vi "plot_isoteric_chart.vi"(7 "W-Array in kg/kg (Input)":dbl[](array[numeric])=[0.01, 0.025, 0.1, 0.2, 0.3, 0.4, 0.5], 8 "Error (Input)":errorcluster, 9 "T_max in K (Input)":dbl=647.0, 10 "T_min in K (Input)":dbl=283.15, 11 "WorkingPair (Input)":T1={"no_iso"=1, "no_p_sat"=1, "path_db"="D:\\Driesel\\SorpLibLocal\\labview_wrapper\\data\\json\\sorpproplib.json", "wp_as"="silica gel pellet", "wp_st"="123", "wp_iso"="DubininArctan1", "wp_rf"="Water", "rf_rhol"="SaturatedLiquidDensity_EoS1", "no_rhol"=1, "rf_psat"="VaporPressure_EoS1"}) -> (0 "Error (Output)":errorcluster, 3 "Isosteres":cluster{dbl[], dbl[]}[](graph)=[{array[365 elements], array[365 elements]}, {array[365 elements], array[365 elements]}, {array[365 elements], array[365 elements]}, {array[365 elements], array[365 elements]}, {array[359 elements], array[359 elements]}, {array[289 elements], array[289 elements]}, {[-0.003531696980399082, -0.0035192679922576107, -0.0035069261792039282, -0.003494670627293378, -0.0034825004353125546, -0.00347041471455839, -0.003458412588621823, -0.0034464931931759437, -0.0034346556757685045, -0.0034228991956186893, -0.003411222923418046, -0.0033996260411354754, -0.0033881077418261903, -0.0033766672294445383, -0.0033653037186606094, -0.0033540164346805303, -0.003342804613070366, -0.003331667499583542, -0.003320604349991699, -0.0033096144299189145, -0.003298697014679202, -0.003287851389117212, -0.003277076847452073, -0.003266372693124286, -0.003255738238645613, -0.0032451728054518907, -0.0032346757237586934, -0.003224246332419797, -0.003213883978788366, -0.0032035880185808108, -0.003193357815743254, -0.0031831927423205475, -0.0031730921783277807, -0.003163055511624229, -0.0031530821377896896, -0.0031431714600031434, -0.0031333228889237038, -0.003123535842573794, -0.0031138097462245057, -0.003104144032283098, -0.0030945381401825778, -0.0030849915162733305, -0.0030755036137167465, -0.0030660738923808067, -0.0030567018187375823, -0.0030473868657626088, -0.0030381285128360932, -0.003028926245645919, -0.0030197795560924054, -0.0030106879421947915, -0.0030016509079994, -0.002992667963489451, -0.002983738624496494, -0.002974862412613417, -0.002966038855109002, -0.0029572674848440043, -0.0029485478401887074, -0.0029398794649419377, -0.0029312619082515023, -0.0029226947245360223, -0.002914177473408131, -0.002905709719599012, -0.0028972910328842532, -0.0028889209880109783, -0.0028805991646262425, -0.002872325147206664, -0.0028640985249892598, -0.00285591889190347, -0.002847785846504343, -0.002839698991906858, -0.002831657935721365, -0.002823662289990117, -0.002815711671124877, -0.002807805699845571, -0.0027999440011199778, -0.002792126204104426, -0.00278435194208548, -0.0027766208524226017, -0.0027689325764917627, -0.0027612867596299878, -0.002753683051080821, -0.002746121103940684, -0.002738600575106121, -0.0027311211252219036, -0.0027236824186299877, -0.0027162841233192994, -0.0027089259108763375, -0.00270160745643658, -0.00269432843863667, -0.002687088539567379, -0.0026798874447273215, -0.0026727248429774158, -0.0026656004264960682, -0.0026585138907350794], [995.6868807653667, 1065.5938991149683, 1139.8574391068994, 1218.7117814882488, 1302.401645095998, 1391.1825454296695, 1485.3211613320625, 1585.0957098471665, 1690.7963293242678, 1802.7254708382966, 1921.1982979968375, 2046.5430952054487, 2179.1016844642027, 2319.229850770136, 2467.297776201945, 2623.690482765518, 2788.808284081765, 2963.067246000752, 3146.899656229439, 3340.7545030642627, 3545.0979633235356, 3760.4138995790445, 3987.2043667916496, 4225.990128460064, 4477.311182398888, 4741.727296267391, 5019.818552977553, 5312.185906117583, 5619.451745534454, 5942.260473227631, 6281.279089715428, 6637.197791044433, 7010.730576623637, 7402.615868075008, 7813.6171393044415, 8244.523558008743, 8696.150638848858, 9169.34090853134, 9664.964583056706, 10183.920257407988, 10727.135607969129, 11295.568107981539, 11890.205756363213, 12512.067820236784, 13162.205591531703, 13841.703158047952, 14551.678189391017, 15293.282738212663, 16067.704057216224, 16876.165432412705, 17719.927033141066, 18600.286779396734, 19518.581227041646, 20476.186471504287, 21474.519070609156, 22515.036987215448, 23599.240552378036, 24728.673449789396, 25904.923722296717, 27129.624801339716, 28404.456560195467, 29731.146391970313, 31111.470313326685, 32547.25409499115, 34040.37442014383, 35592.76007185284, 37206.393150778495, 38883.310324442566, 40625.60410942416, 42435.42418792465, 44314.97876021472, 46266.53593457144, 48292.42515638591, 50395.03867823235, 52576.83307276827, 54840.33079046082, 57188.121764219315, 59622.8650631532, 62147.29059777922, 64764.20087914201, 67476.47283444299, 70287.0596819237, 73198.99286789467, 76215.38406897619, 79339.42726277668, 82574.40087043002, 85923.66997459781, 89390.68861675632, 92979.00217780344, 96692.2498462531, 100534.16717853813, 104508.58875619763, 108619.45094501246, 112870.79476144738]}, {[], []}])   [LabVIEW 2017]
panel:
  out "ID of temperature loop":i32=364
  # "Path to database"
  # "Name of sorbent"
  # "Name of sub-type of sorbent"
  # "Name of refrigerant"
  # "Name of isotherm"
  # "ID of isotherm"
  # "Name of calculation approach for vapor pressure"
  # "ID of vapor pressure equation"
  # "Name of calculation approach for liquid density"
  # "ID of liquid density equation"
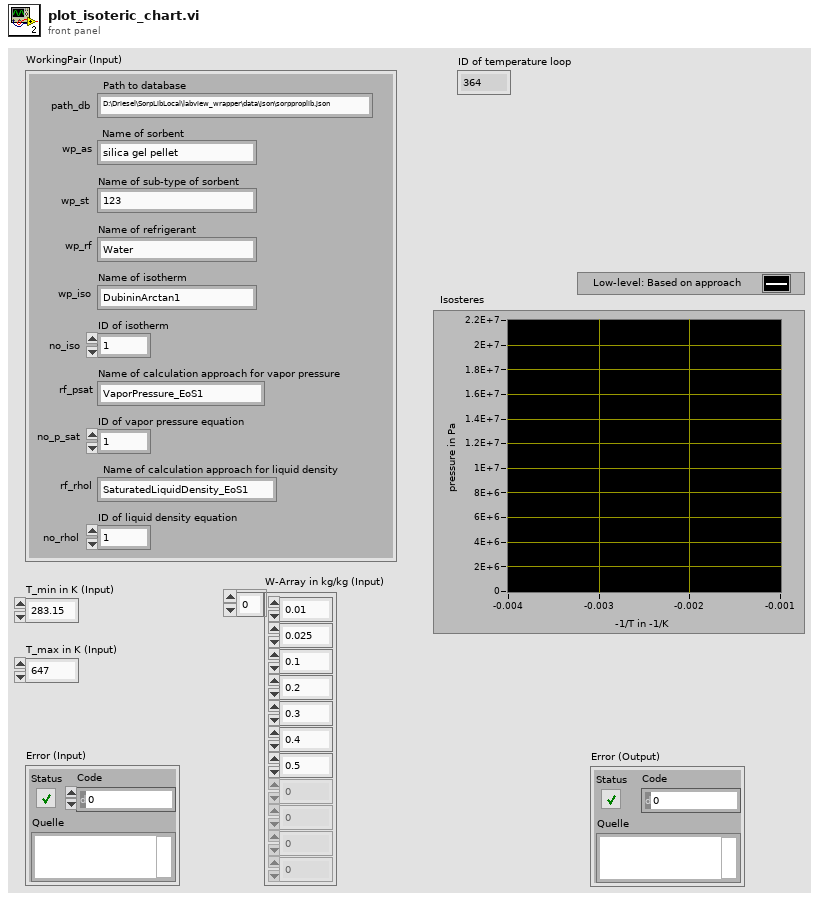
[diagram p1: front panel]
types:
  T1 = cluster{"no_iso":i32, "no_p_sat":i32, "path_db":string, "wp_as":string, "wp_st":string, "wp_iso":string, "wp_rf":string, "rf_rhol":string, "no_rhol":i32, "rf_psat":string}
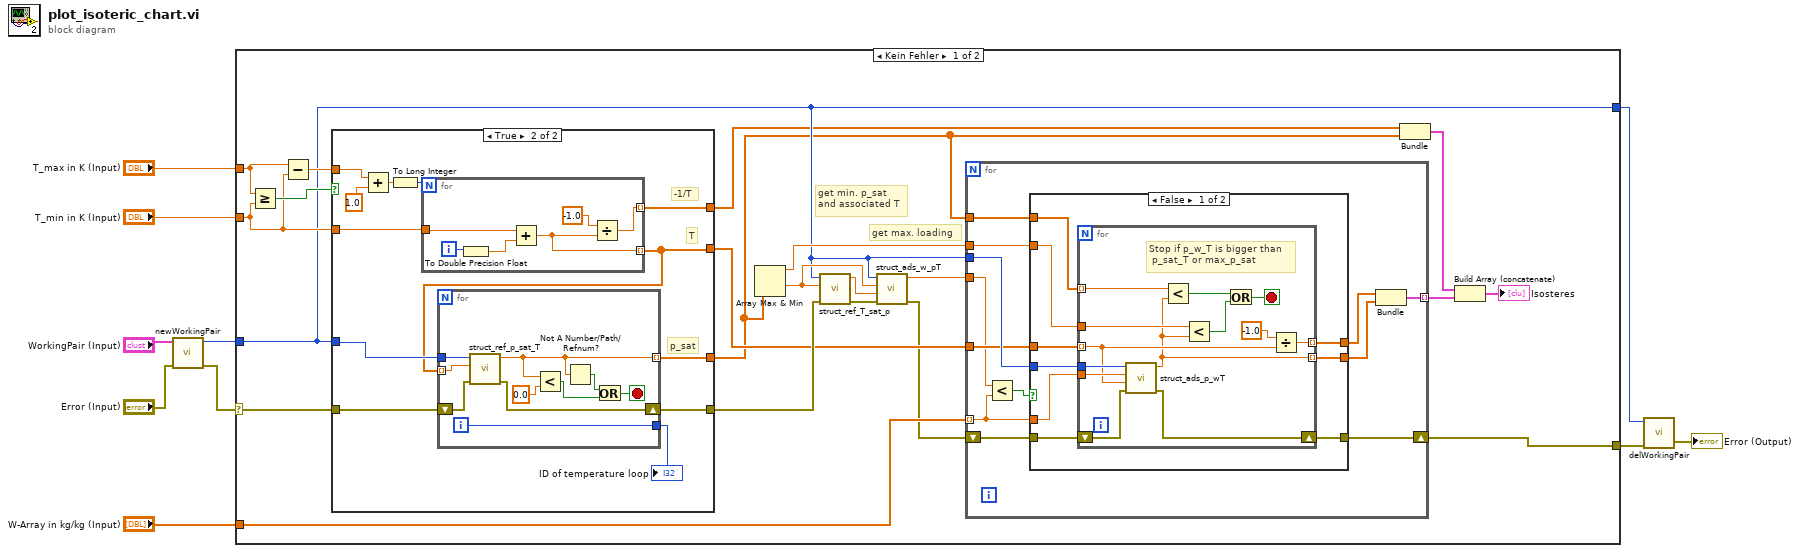
[diagram p0: block diagram]
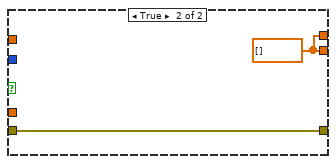
[diagram p2: hidden frame]
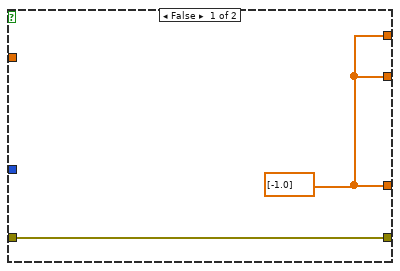
[diagram p3: hidden frame]
diagram:
  n1 = call "newWorkingPair.vi"("Error (Input)"="Error (Input)", "WorkingPair (Input)"="WorkingPair (Input)") -> ("Error (Output)"=w7:errorcluster, "workingPair"=w5:i64)  [unwired: 8 in]
  n2 = case shown="Kein Fehler" w7 {
    selector: w7 -> [w27 w99]
    tunnel: [w22 w99] -> w2
    tunnel: "T_min in K (Input)" -> [w28 _]
    tunnel: "T_max in K (Input)" -> [w30 _]
    tunnel: w5 -> [w14 w98]
    tunnel: "W-Array in kg/kg (Input)" -> [w25 _]
    tunnel: [w14 w98] -> w3
    frame No Error {
      # "get max. loading"
      # "get min. p_sat \nand associated T"
      n3 = Greater Or Equal?(x=w30, y=w28) -> (x >= y?=w31:bool)
      n4 = Subtract(x=w30, y=w28) -> (x-y=w29:dbl)
      n5 = case shown="True" w31 {
        tunnel: w29 -> [_ w72]
        tunnel: w28 -> [_ w81]
        tunnel: [w68 w78] -> w24
        tunnel: w27 -> [w69 w77]
        tunnel: w14 -> [_ w80]
        tunnel: [w68 w79] -> w11
        tunnel: [w68 w75] -> w13
        tunnel: [w69 w74] -> w26
        frame False {
          w68 = dbl[] [-1.0]
        }
        frame True {
          # "p_sat"
          # "T"
          # "-1/T"
          n6 = Add(x=w72, y=1.0) -> (x+y=w70:dbl)
          n7 = To Long Integer(number=w70) -> (32bit integer=w73:i32)
          n8 = for {
            N: w73 -> [_]
            tunnel: w81 -> [w97]
            tunnel: [w93] -> w78 mode=indexing
            tunnel: [w92] -> w75 mode=indexing
            i -> [w96]
            n9 = To Double Precision Float(number=w96) -> (double precision float=w95:dbl)
            n10 = Add(x=w97, y=w95) -> (x+y=w93:dbl)
            n11 = Divide(x=-1.0, y=w93) -> (x/y=w92:dbl)
          }
          n12 = for {
            tunnel: w78 -> [w88] mode=indexing
            tunnel: w80 -> [w90]
            tunnel: [w83] -> w79 mode=indexing
            shift-right: [w89] -> w74
            shift-left: w77 -> [w91]
            tunnel: [w87] -> w76
            i -> [w87]
            stop <- w84 stop-if-true
            n13 = call "struct_ref_p_sat_T.vi"("Error (Input)"=w91, "Temperature in K (Input)"=w88, "Reference working pair (Input)"=w90) -> ("Error (Output)"=w89:errorcluster, "Saturation pressure in Pa (Output)"=w83:dbl)  [unwired: 7 in]
            n14 = Less?(x=w83, y=0.0) -> (x < y?=w85:bool)
            n15 = Not A Number/Path/Refnum?(number/path/refnum=w83) -> (NaN/Path/Refnum?=w82:bool)
            n16 = Or(x=w82, y=w85) -> (x .or. y?=w84:bool)
          }
          "ID of temperature loop" <- w76
        }
      }
      n17 = Array Max & Min(array=w11) -> (max value=w23:dbl, min value=w18:dbl)  [unwired: 2 out]
      n18 = call "struct_ref_T_sat_p.vi"("Error (Input)"=w26, "Saturation pressure in Pa (Input)"=w18, "Reference working pair (Input)"=w14) -> ("Error (Output)"=w20:errorcluster, "Temperature in K (Output)"=w19:dbl)  [unwired: 7 in]
      n19 = call "struct_ads_w_pT.vi"("Error (Input)"=w20, "Temperature in K (Input)"=w19, "Pressure in Pa (Input)"=w18, "Reference working pair (Input)"=w14) -> ("Error (Output)"=w21:errorcluster, "Loading in kg/kg (Output)"=w17:dbl)  [unwired: 6 in]
      n20 = for {
        tunnel: w25 -> [w34] mode=indexing
        tunnel: w14 -> [w42]
        tunnel: w24 -> [w41]
        tunnel: w11 -> [w40]
        tunnel: w23 -> [w39]
        tunnel: [w38] -> w16 mode=indexing
        shift-right: [w37] -> w22
        shift-left: w21 -> [w43]
        tunnel: w17 -> [w35]
        n21 = Less?(x=w35, y=w34) -> (x < y?=w33:bool)
        n22 = case shown="False" w33 {
          tunnel: w43 -> [w52 w67]
          tunnel: w42 -> [w51 _]
          tunnel: w41 -> [w50 _]
          tunnel: w40 -> [w49 _]
          tunnel: w39 -> [w48 _]
          tunnel: [w47 w67] -> w37
          tunnel: [w46 w66] -> w36
          tunnel: w34 -> [w45 _]
          tunnel: [w44 w66] -> w32
          frame False {
            n23 = for {
              tunnel: w45 -> [w64]
              tunnel: w51 -> [w63]
              tunnel: w50 -> [w57] mode=indexing
              tunnel: w49 -> [w59] mode=indexing
              shift-right: [w62] -> w47
              shift-left: w52 -> [w65]
              tunnel: w48 -> [w61]
              tunnel: [w53] -> w46 mode=indexing
              tunnel: [w56] -> w44 mode=indexing
              stop <- w60 stop-if-true
              # "Stop if p_w_T is bigger than\n p_sat_T or max_p_sat"
              n24 = call "struct_ads_p_wT.vi"("Error (Input)"=w65, "Temperature in K (Input)"=w57, "Loading in kg/kg (Input)"=w64, "Reference working pair (Input)"=w63) -> ("Error (Output)"=w62:errorcluster, "Pressure in Pa (Output)"=w53:dbl)  [unwired: 6 in]
              n25 = Less?(x=w59, y=w53) -> (x < y?=w54:bool)
              n26 = Less?(x=w61, y=w53) -> (x < y?=w55:bool)
              n27 = Or(x=w54, y=w55) -> (x .or. y?=w60:bool)
              n28 = Divide(x=-1.0, y=w57) -> (x/y=w56:dbl)
            }
          }
          frame True {
            w66 = dbl[] []
          }
        }
        n29 = Bundle(w32, w36) -> (w38:cluster{dbl[], dbl[]})  [unwired: 1 in]
      }
      n30 = Bundle(w13, w11) -> (w12:cluster{dbl[], dbl[]})  [unwired: 1 in]
      n31 = Build Array (concatenate)(w12, w16) -> (→"Isosteres":cluster{dbl[], dbl[]}[])
    }
    frame Error {
    }
  }
  n32 = call "delWorkingPair.vi"("Error (Input)"=w2, "workingPair"=w3) -> ("Error (Output)"=→"Error (Output)":errorcluster)  [unwired: 9 in]
